vi "Test All Levels.vi"() -> ()   [LabVIEW 2022 SP3]
uses:
  VoiceMeeterRemote/Voicemeeter Type.ctl
  VoiceMeeterRemote/VoiceMeeterRemote/VoiceMeeterRemote.lvclass
  VoiceMeeterRemote/VoiceMeeterRemote.lvlib
panel:
  out "Type":T1
  in  "stop":bool
  out "Levels":sgl[](array[slide]) scale=0.0..1.0
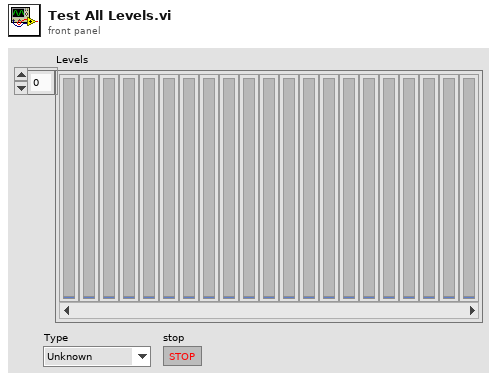
[diagram p1: front panel]
types:
  T1 = typedef "VoiceMeeterRemote.lvlib/Voicemeeter Type.ctl" = enum16{"Unknown", "Voicemeeter", "Banana", "Potato", "Potato x64"}
  T2 = typedef "VoiceMeeterRemote.lvlib/Levels.ctl" = cluster{"Input Pre Fader":T3[], "Input Post Fader":T3[], "Input Post Mute":T3[], "Output":T3[]}
  T3 = typedef "VoiceMeeterRemote.lvlib/Device Channels.ctl" = cluster{"Values":sgl[]}
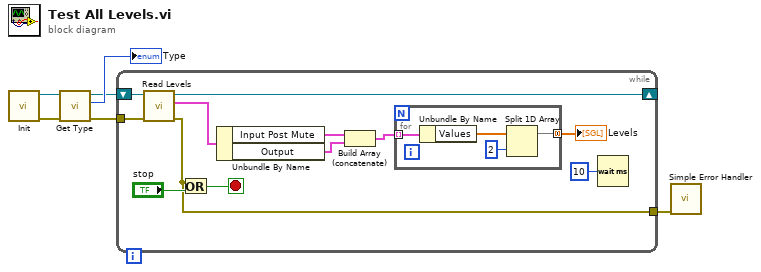
[diagram p0: block diagram]
diagram:
  n1 = call "Init.vi"() -> ("error out"=w3:errorcluster, "VoiceMeeterRemote out"=w6:refnum<class "VoiceMeeterRemote.lvclass">)  [unwired: 9 in, 1 out]
  n2 = call "Get Type.vi"("error in (no error)"=w3, "VoiceMeeterRemote in"=w6) -> ("error out"=w2:errorcluster, "Type"=→"Type":T1, "VoiceMeeterRemote out"=w4:refnum<class "VoiceMeeterRemote.lvclass">)  [unwired: 7 in]
  n3 = while {
    shift-right: [w16] -> _
    shift-left: w4 -> [w18]
    tunnel: w2 -> [w10]
    tunnel: [w7] -> w1
    stop <- w9 stop-if-true
    n4 = call "Read Levels.vi"("error in (no error)"=w10, "VoiceMeeterRemote in"=w18) -> ("error out"=w7:errorcluster, "Levels"=w15:T2, "VoiceMeeterRemote out"=w16:refnum<class "VoiceMeeterRemote.lvclass">)  [unwired: 7 in]
    n5 = Or(x=w7, y="stop") -> (x .or. y?=w9:bool)
    n6 = Unbundle By Name(w15) -> ("Input Post Mute"=w14:T3[], "Output"=w11:T3[])
    n7 = Build Array (concatenate)(w14, w11) -> (w12:T3[])
    n8 = for {
      tunnel: w12 -> [w22] mode=indexing
      tunnel: [w19] -> w13 mode=concatenating
      n9 = Unbundle By Name(w22) -> ("Values"=w21:sgl[])
      n10 = Split 1D Array(array=w21, index=2) -> (first subarray=w19:sgl[])  [unwired: 1 out]
    }
    "Levels" <- w13
    n11 = Wait (ms)(milliseconds to wait=u32 10) -> ()  [unwired: 1 out]
  }
  n12 = call <vilib>:"Simple Error Handler.vi"("error in (no error)"=w1) -> ()  [unwired: 4 in, 5 out]
